vi "ExpandAndLinkNodes.vi"(8 "error in (no error)":errorcluster, 10 "ToExpand in":refnum<data-value>, 11 "MultiTree in":refnum<class "MultiTree.lvclass">) -> (0 "error out":errorcluster, 1 "ExpandedSearchNodes":refnum<data-value>[](array[refnum]), 2 "ToExpand out":refnum<data-value>, 3 "MultiTree out":refnum<class "MultiTree.lvclass">)   [LabVIEW 2014, in "MultiTree.lvlib" / "MultiTree.lvclass"]
uses:
  <userlib>/AdvancedDataStructures/ClassBased/MultiTree/MultiTree.lvclass
  <userlib>/AdvancedDataStructures/ClassBased/MultiTreeNode/MultiTreeNode.lvclass
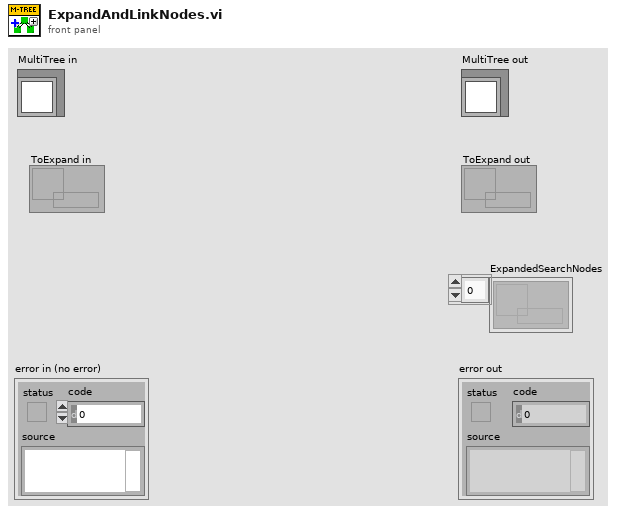
[diagram p1: front panel]
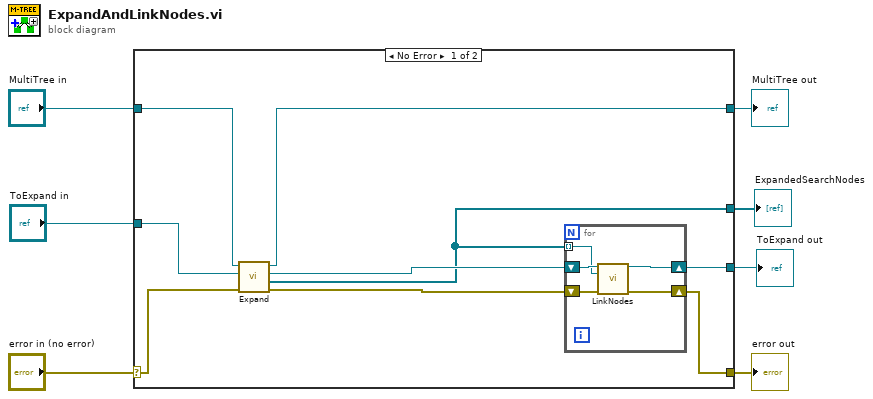
[diagram p0: block diagram]
diagram:
  n1 = case shown="No Error" "error in (no error)" {
    selector: "error in (no error)" -> [w11 w24]
    tunnel: [w8 w24] -> w6
    tunnel: [w13 w23] -> w4
    tunnel: "MultiTree in" -> [w14 w23]
    tunnel: "ToExpand in" -> [w12 w22]
    tunnel: [w10 _] -> w2
    tunnel: [w9 w22] -> w1
    frame No Error {
      n2 = call-dynamic "Expand.vi"("error in (no error)"=w11, "ToExpand in"=w12, "MultiTree in"=w14) -> ("error out"=w15:errorcluster, "ExpandedSearchNodes"=w10:refnum<data-value>[], "ToExpand out"=w16:refnum<data-value>, "MultiTree out"=w13:refnum<class "MultiTree.lvclass">)  [unwired: 5 in]
      n3 = for {
        shift-right: [w19] -> w8
        shift-left: w15 -> [w20]
        tunnel: w10 -> [w18] mode=indexing
        shift-right: [w17] -> w9
        shift-left: w16 -> [w21]
        n4 = call <userlib>:"LinkNodes.vi"("Parent in"=w21, "Child in"=w18, "error in (no error)"=w20) -> ("Parent out"=w17:refnum<data-value>, "error out"=w19:errorcluster)  [unwired: 10 in, 1 out]
      }
    }
    frame Error {
    }
  }
  "error out" <- w6
  "MultiTree out" <- w4
  "ToExpand out" <- w1
  "ExpandedSearchNodes" <- w2
